vi "Generate Data.vi"(8 "entrée d'erreur":errorcluster, 11 "Nombre de voies":i32) -> (0 "sortie d'erreur":errorcluster, 2 "Spectre de puissance":waveform(dbl)[](graph), 3 "Graphe déroulant":waveform(dbl)[](graph))   [LabVIEW 2009]
uses:
  Instance           4 21Saved   Generate Data .vi
  Instance           3 21Saved   Generate Data .vi
  <vilib>/express/express analysis/Spectral/XNode/ExpressSpectralMeasurementsBlockNode.xnode
  <vilib>/express/express analysis/Spectral/Block/exnSpectralBlock spectral measurements power poly.vi
  <vilib>/express/express analysis/Spectral/Block/exnSpectralBlock spectral measurements power DDT.vi
panel:
  in  "Vide":dynamicdata(waveform)
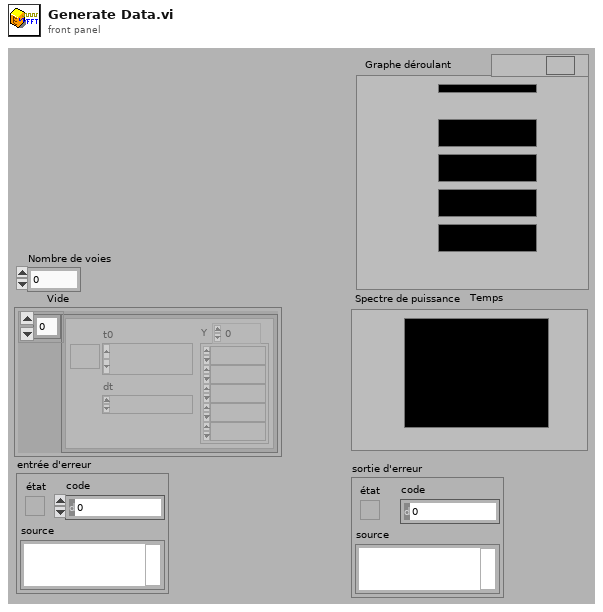
[diagram p1: front panel]
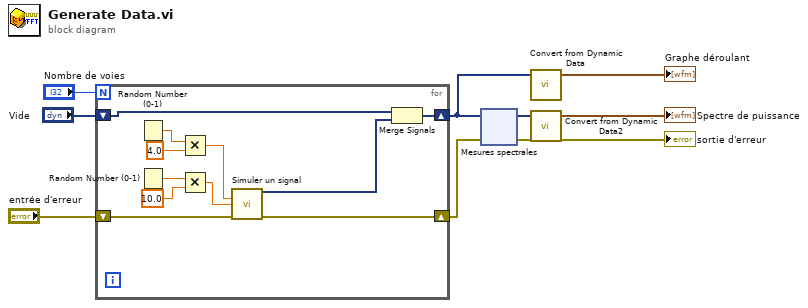
[diagram p0: block diagram]
diagram:
  n1 = for "Boucle For" {
    N: "Nombre de voies" -> [_]
    shift-right: [w14] -> w7
    shift-left: "entrée d'erreur" -> [w18]
    shift-right: [w17] -> w5
    shift-left: "Vide" -> [w15]
    n2 = Random Number (0-1) ("Nombre aléatoire (0-1)")() -> (number: 0 to 1=w12:dbl)
    n3 = Random Number (0-1) ("Nombre aléatoire (0-1)")() -> (number: 0 to 1=w20:dbl)
    n4 = Multiply ("Multiplier")(x=w12, y=4.0) -> (x*y=w11:dbl)
    n5 = Multiply ("Multiplier")(x=w20, y=10.0) -> (x*y=w10:dbl)
    n6 = call "Simuler un signal"("Frequency"=w11, "Amplitude"=w10, "error in (no error)"=w18) -> ("Sinus"=w16:dynamicdata, "error out"=w14:errorcluster)  [unwired: 11 in]
    n7 = Merge Signals ("Assembler des signaux")(w15, w16) -> (w17:dynamicdata)
  }
  n8 = xnode "Mesures spectrales"("Signaux"=w5, "entrée d'erreur (pas d'erreur)"=w7) -> ("Spectre de puissance"=w3:dynamicdata, "sortie d'erreur"=→"sortie d'erreur":errorcluster)
  n9 = call "Convert from Dynamic Data"("Dynamic Data Type"=w5) -> ("Array of Waveform"=→"Graphe déroulant":waveform(dbl)[])  [unwired: 3 in]
  n10 = call "Convert from Dynamic Data2"("Dynamic Data Type"=w3) -> ("Array of Waveform"=→"Spectre de puissance":waveform(dbl)[])  [unwired: 3 in]
